vi "BalancingBallPID.vi"() -> ()   [LabVIEW 2020]
uses:
  <vilib>/MakerHub/LINX/Public/Utilities/Open Serial.vi
  <vilib>/MakerHub/LINX/Public/Sensors/Motion/Servo/Servo Open One Channel.vi
  <vilib>/addons/control/pid/pid.llb/PID (DBL).vi
  <vilib>/MakerHub/LINX/Public/Sensors/Motion/Servo/Servo Close One Channel.vi
  <vilib>/MakerHub/LINX/LMH-LINX.lvlib
  <vilib>/MakerHub/LINX/Public/Sensors/Motion/Servo/Servo.lvlib
  <vilib>/MakerHub/LINX/Public/Sensors/Distance/Ultrasonic/Ultrasonic.lvlib
  <vilib>/addons/control/pid/NI_PID_pid.lvlib
panel:
  in  "median filter order":i32=2
  in  "angle_mid_point":dbl
  in  "PID":bool
  in  "Angle Range":cluster{"output high":dbl, "output low":dbl}={"output high"=100.0, "output low"=-100.0} {"output low" format="%.2f"; "output high" format="%.2f"}
  in  "target":dbl(slide) scale=0.0..42.0
  in  "PID gains":T1={"proportional gain (Kc)"=1.0, "integral time (Ti, min)"=0.01, "derivative time (Td, min)"=0.0} {"derivative time (Td, min)" format="%.3f"; "integral time (Ti, min)" format="%.3f"; "proportional gain (Kc)" format="%.3f"}
  in  "Manual Control":dbl(knob) scale=0.0..180.0
  in  "stop":bool
  out "Position Error":cluster{dbl, i32}(graph)
  # "target: Η απόσταση από τον αισθητήρα που θέλουμε να ισορροπήσει το μπαλάκι.\nPID gains : Τα κέρδη του PID ελεγκτή.\nAngle_mid_point : Η γωνία εισόδου στο servo ώστε η ράβδος να είναι παράλληλη με το έδαφος.\nAngle Range: Το εύρος γωνιών (σε σχέση με το angle_mid_point) που δίνει ως έξοδο ο PID ελεγκτής.\nMedian filter order: Η τάξη του median φίλτρου που εξομαλύνει τις τιμές του αισθητήρα.\nPID control on/off: Ενεργοποιεί ή απενεργοποιεί τον PID ελεγκτή.\nManual Control : Σε περίπτωση που είναι απενεργοποιημένος ο PID ελεγκτής ορίζεται απευθείας η γωνία στο servo"
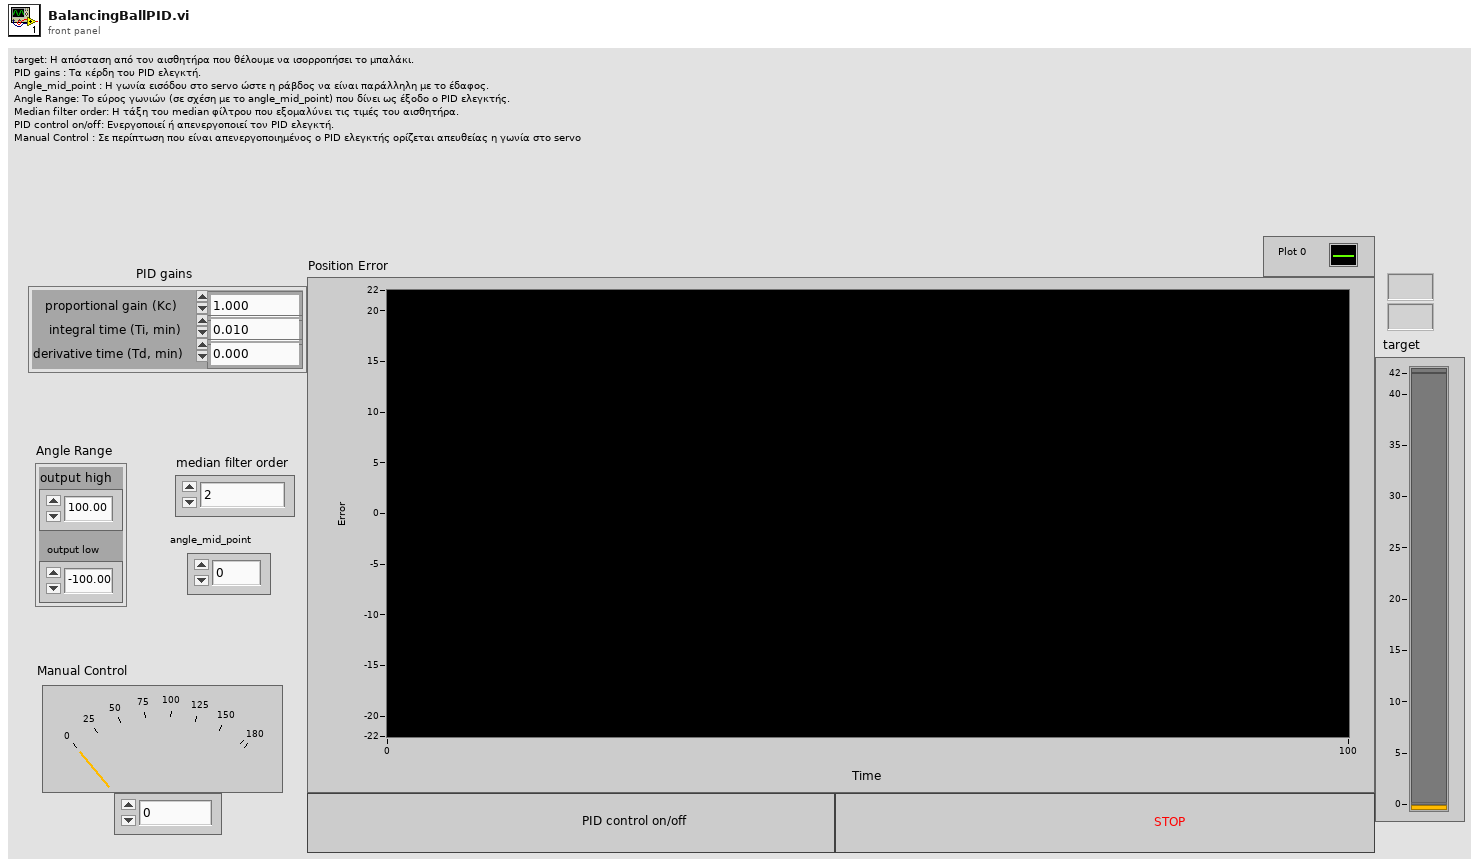
[diagram p1: front panel]
types:
  T1 = cluster{"proportional gain (Kc)":dbl, "integral time (Ti, min)":dbl, "derivative time (Td, min)":dbl}
  T2 = typedef "LMH-LINX.lvlib/LINX Ref.ctl" = cluster{"IO":T3, "Interface":T4, "LINX Device Config":T5}
  T3 = typedef "LMH-LINX.lvlib/Platform.ctl" = enum16{"Remote", "Local"}
  T4 = typedef "LMH-LINX.lvlib/Interface.ctl" = enum16{"Serial", "TCP"}
  T5 = typedef "LMH-LINX.lvlib/Device.lvlib/LINX Device Config.ctl" = cluster{"Interface":T4, "COM Port":refnum<visa-resource-name>, "TCP Configuration":T6, "Device Family":u8, "Device ID":u8, "Device Name":string, "TCP Ref":refnum<k5>, "Channels":T7}
  T6 = typedef "LMH-LINX.lvlib/Device.lvlib/TCP Config.ctl" = cluster{"IP Address":string, "Port":u16}
  T7 = typedef "LMH-LINX.lvlib/Channels.ctl" = cluster{"DI":u8[], "DO":u8[], "AI":u8[], "AO":u8[], "PWM":u8[], "QE":u8[], "UART":u8[], "I2C 2":u8[], "SPI":u8[], "CAN":u8[], "Servo":u8[], "AI Ref (V)":dbl, "AI Resolution (Bits)":u8, "AO Ref (V)":dbl, "AO Resolution (Bits)":u8}
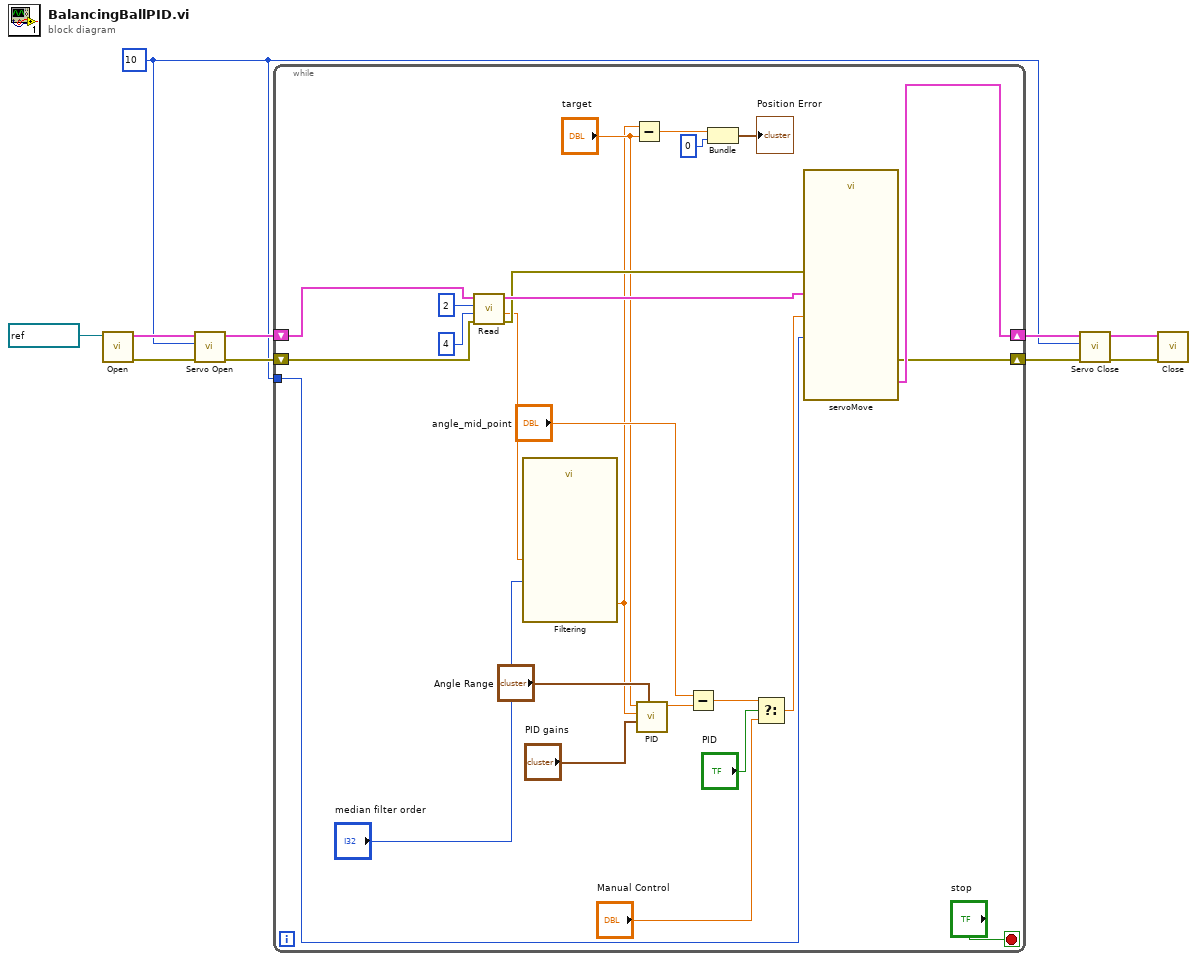
[diagram p0: block diagram]
diagram:
  w1 = u8 10 ("Servo Channel")
  n1 = call-poly <vilib>:"Open.vi"("Serial Port"=refnum<visa-resource-name> "COM3") -> ("Error Out"=w8:errorcluster, "LINX Resource"=w9:T2)  [unwired: 8 in, 1 out]
  n2 = call-poly <vilib>:"Servo Open.vi"("Error In"=w8, "Servo Channel"=w1, "LINX Resource"=w9) -> ("Error Out"=w6:errorcluster, "LINX Resource"=w7:T2)  [unwired: 7 in]
  n3 = while {
    shift-right: [w27] -> w4
    shift-left: w6 -> [w34]
    shift-right: [w28] -> w5
    shift-left: w7 -> [w35]
    tunnel: w1 -> [w26]
    stop <- "stop" stop-if-true
    n4 = call <vilib>:"Read.vi"("Error In"=w34, "DO Channel"=u8 4, "DI Channel"=u8 2, "LINX Resource"=w35) -> ("Error Out"=w29:errorcluster, "Centimeters"=w11:dbl, "LINX Resource"=w30:T2)  [unwired: 4 in, 1 out]
    n5 = call "Filtering.vi"("order"="median filter order", "Centimeters"=w11) -> ("output"=w12:dbl)  [unwired: 9 in]
    n6 = Subtract(x=w12, y="target") -> (x-y=w16:dbl)
    n7 = call-poly <vilib>:"PID.vi"("output range"="Angle Range", "PID gains"="PID gains", "process variable"=w12, "setpoint"="target") -> ("output"=w24:dbl)  [unwired: 6 in, 1 out]
    n8 = Subtract(x="angle_mid_point", y=w24) -> (x-y=w21:dbl)
    n9 = Bundle(w16, 0) -> (→"Position Error":cluster{dbl, i32})  [unwired: 1 in]
    n10 = Select(t=w21, s="PID", f="Manual Control") -> (s? t:f=w20:dbl)
    n11 = call "servoMove.vi"("error in (no error)"=w29, "servo angle"=w20, "LINX Resource in"=w30, "Servo Channel"=w26) -> ("error out"=w27:errorcluster, "LINX Resource out"=w28:T2)  [unwired: 6 in]
  }
  n12 = call-poly <vilib>:"Servo Close.vi"("Error In"=w4, "Servo Channel"=w1, "LINX Resource"=w5) -> ("Error Out"=w2:errorcluster, "LINX Resource"=w3:T2)  [unwired: 7 in]
  n13 = call <vilib>:"Close.vi"("Error In"=w2, "LINX Resource"=w3) -> ()  [unwired: 9 in, 1 out]
